vi "ReloderSteps.vi"   [LabVIEW 2016]
uses:
  Globals/Globals.vi
types:
  T1 = typedef "WPI_DigitalOutputDevRef.ctl" = cluster{"DIO Channel":T2, "DevStatus":errorcluster}
  T2 = typedef "FPGA_DIOChannel.ctl" = enum8{"DIO 0", "DIO 1", "DIO 2", "DIO 3", "DIO 4", "DIO 5", "DIO 6", "DIO 7", "DIO 8", "DIO 9", "DIO MXP 0", "DIO MXP 1", "DIO MXP 2", "DIO MXP 3", "DIO MXP 4", "DIO MXP 5", "DIO MXP 6", "DIO MXP 7", "DIO MXP 8", "DIO MXP 9", "DIO MXP 10", "DIO MXP 11", "DIO MXP 12", "DIO MXP 13", "DIO MXP 14", "DIO MXP 15", "SPI Port CS1", "SPI Port CS2", "SPI Port CS3", "SPI Port MISO", "SPI Port MOSI", "Invalid"}
  T3 = typedef "WPI_ServoDeviceRef.ctl" = cluster{"DeviceStatus":errorcluster, "PWM Channel":T4, "DeadBand":T5}
  T4 = typedef "FPGA_DIOPWMChannel.ctl" = enum8{"PWM 0", "PWM 1", "PWM 2", "PWM 3", "PWM 4", "PWM 5", "PWM 6", "PWM 7", "PWM 8", "PWM 9", "PWM MXP 0", "PWM MXP 1", "PWM MXP 2", "PWM MXP 3", "PWM MXP 4", "PWM MXP 5", "PWM MXP 6", "PWM MXP 7", "PWM MXP 8", "PWM MXP 9", "Invalid"}
  T5 = typedef "WPI_PWMDeadband.ctl" = cluster{"Name":string, "maxPositivePwm":i32, "minPositivePwm":i32, "centerPwm":i32, "maxNegativePwm":i32, "minNegativePwm":i32, "angularRange":u16}
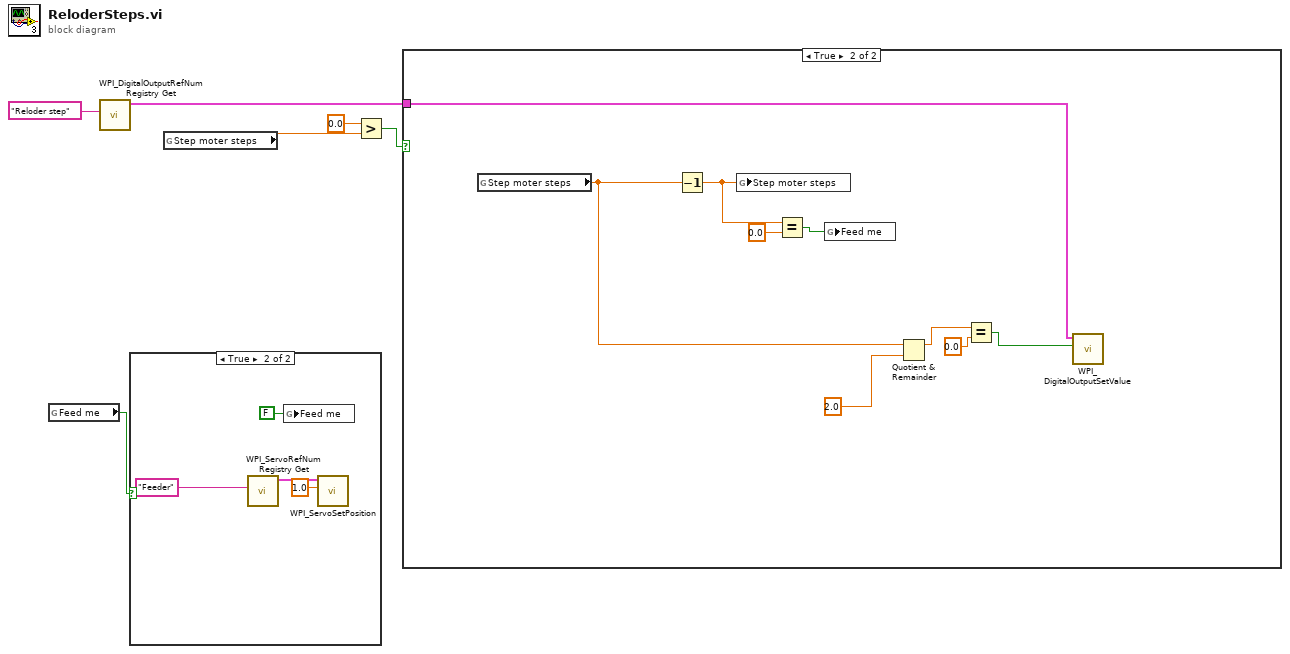
[diagram p0: block diagram]
diagram:
  n1 = global read "Globals.vi" "Feed me"() -> (w1:bool)
  n2 = call <vilib>:"WPI_DigitalOutputRefNum Registry Get.vi"("refnum name"="Reloder step") -> ("DigitalOutputDevRef"=w2:T1)  [unwired: 9 in, 1 out]
  n3 = case shown="True" w1 {
    frame False {
    }
    frame True {
      n4 = call <vilib>:"WPI_ServoRefNum Registry Get.vi"("refnum name"="Feeder") -> ("ServoDeviceRef"=w9:T3)  [unwired: 9 in, 1 out]
      n5 = global write "Globals.vi" "Feed me"(FALSE ("Feed me")) -> ()
      n6 = call <vilib>:"WPI_ServoSetPosition.vi"("Position"=1.0, "ServoDeviceRef"=w9) -> ()  [unwired: 8 in, 2 out]
    }
  }
  n7 = global read "Globals.vi" "Step moter steps"() -> (w5:dbl)
  n8 = Greater?(x=0.0, y=w5) -> (0:w3:bool)
  n9 = case shown="True" w3 {
    tunnel: w2 -> [_ w14]
    frame False {
    }
    frame True {
      n10 = global read "Globals.vi" "Step moter steps"() -> (w19:dbl)
      n11 = Decrement(x=w19) -> (x-1=w13:dbl)
      n12 = global write "Globals.vi" "Step moter steps"(w13) -> ()
      n13 = Equal?(x=w13, y=0.0) -> (x = y?=w11:bool)
      n14 = global write "Globals.vi" "Feed me"(w11) -> ()
      n15 = Quotient & Remainder(x=w19, y=2.0) -> (x-y*floor(x/y)=w17:dbl)  [unwired: 1 out]
      n16 = Equal?(x=w17, y=0.0) -> (x = y?=w15:bool)
      n17 = call <vilib>:"WPI_DigitalOutputSetValue.vi"("Value"=w15, "DigitalOutputDevRef"=w14) -> ()  [unwired: 8 in, 2 out]
    }
  }
